vi "filled buttons.vi"(9 "control-level":string, 11 "Material-Scheme in":refnum<class "Material-Scheme.lvclass">) -> (1 "font color":u32(colorbox), 2 "colors array":cluster{"bg":u32, "fg":u32}[](array[cluster]))   [LabVIEW 2021, in "TSC Material Theme.lvlib" / "Material-Scheme.lvclass"]
doc: "application of the FILLED buttons coloring rules\n\nhttps://m3.material.io/components/buttons/specs#7b9ba06e-d393-491b-830e-ae3fe0816d4b\n\n<b>Code Developed By:</b> +\nDaniel Coons +\nTechnology Service Corporation +\nwww.tsc.com/atcs"
uses:
  Material-Scheme.lvclass
  Material-Scheme.lvclass/Material-Scheme.ctl
  <vilib>/Utility/colorconv.llb/Color to RGB.vi
  <vilib>/Utility/colorconv.llb/RGB to Color.vi
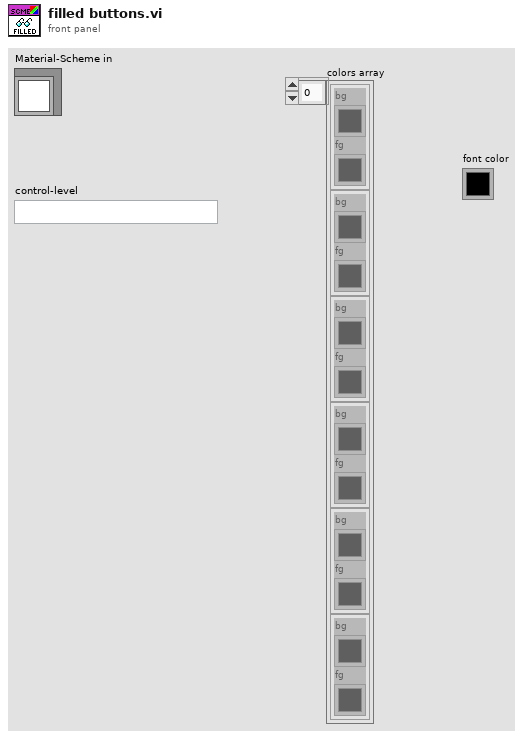
[diagram p1: front panel]
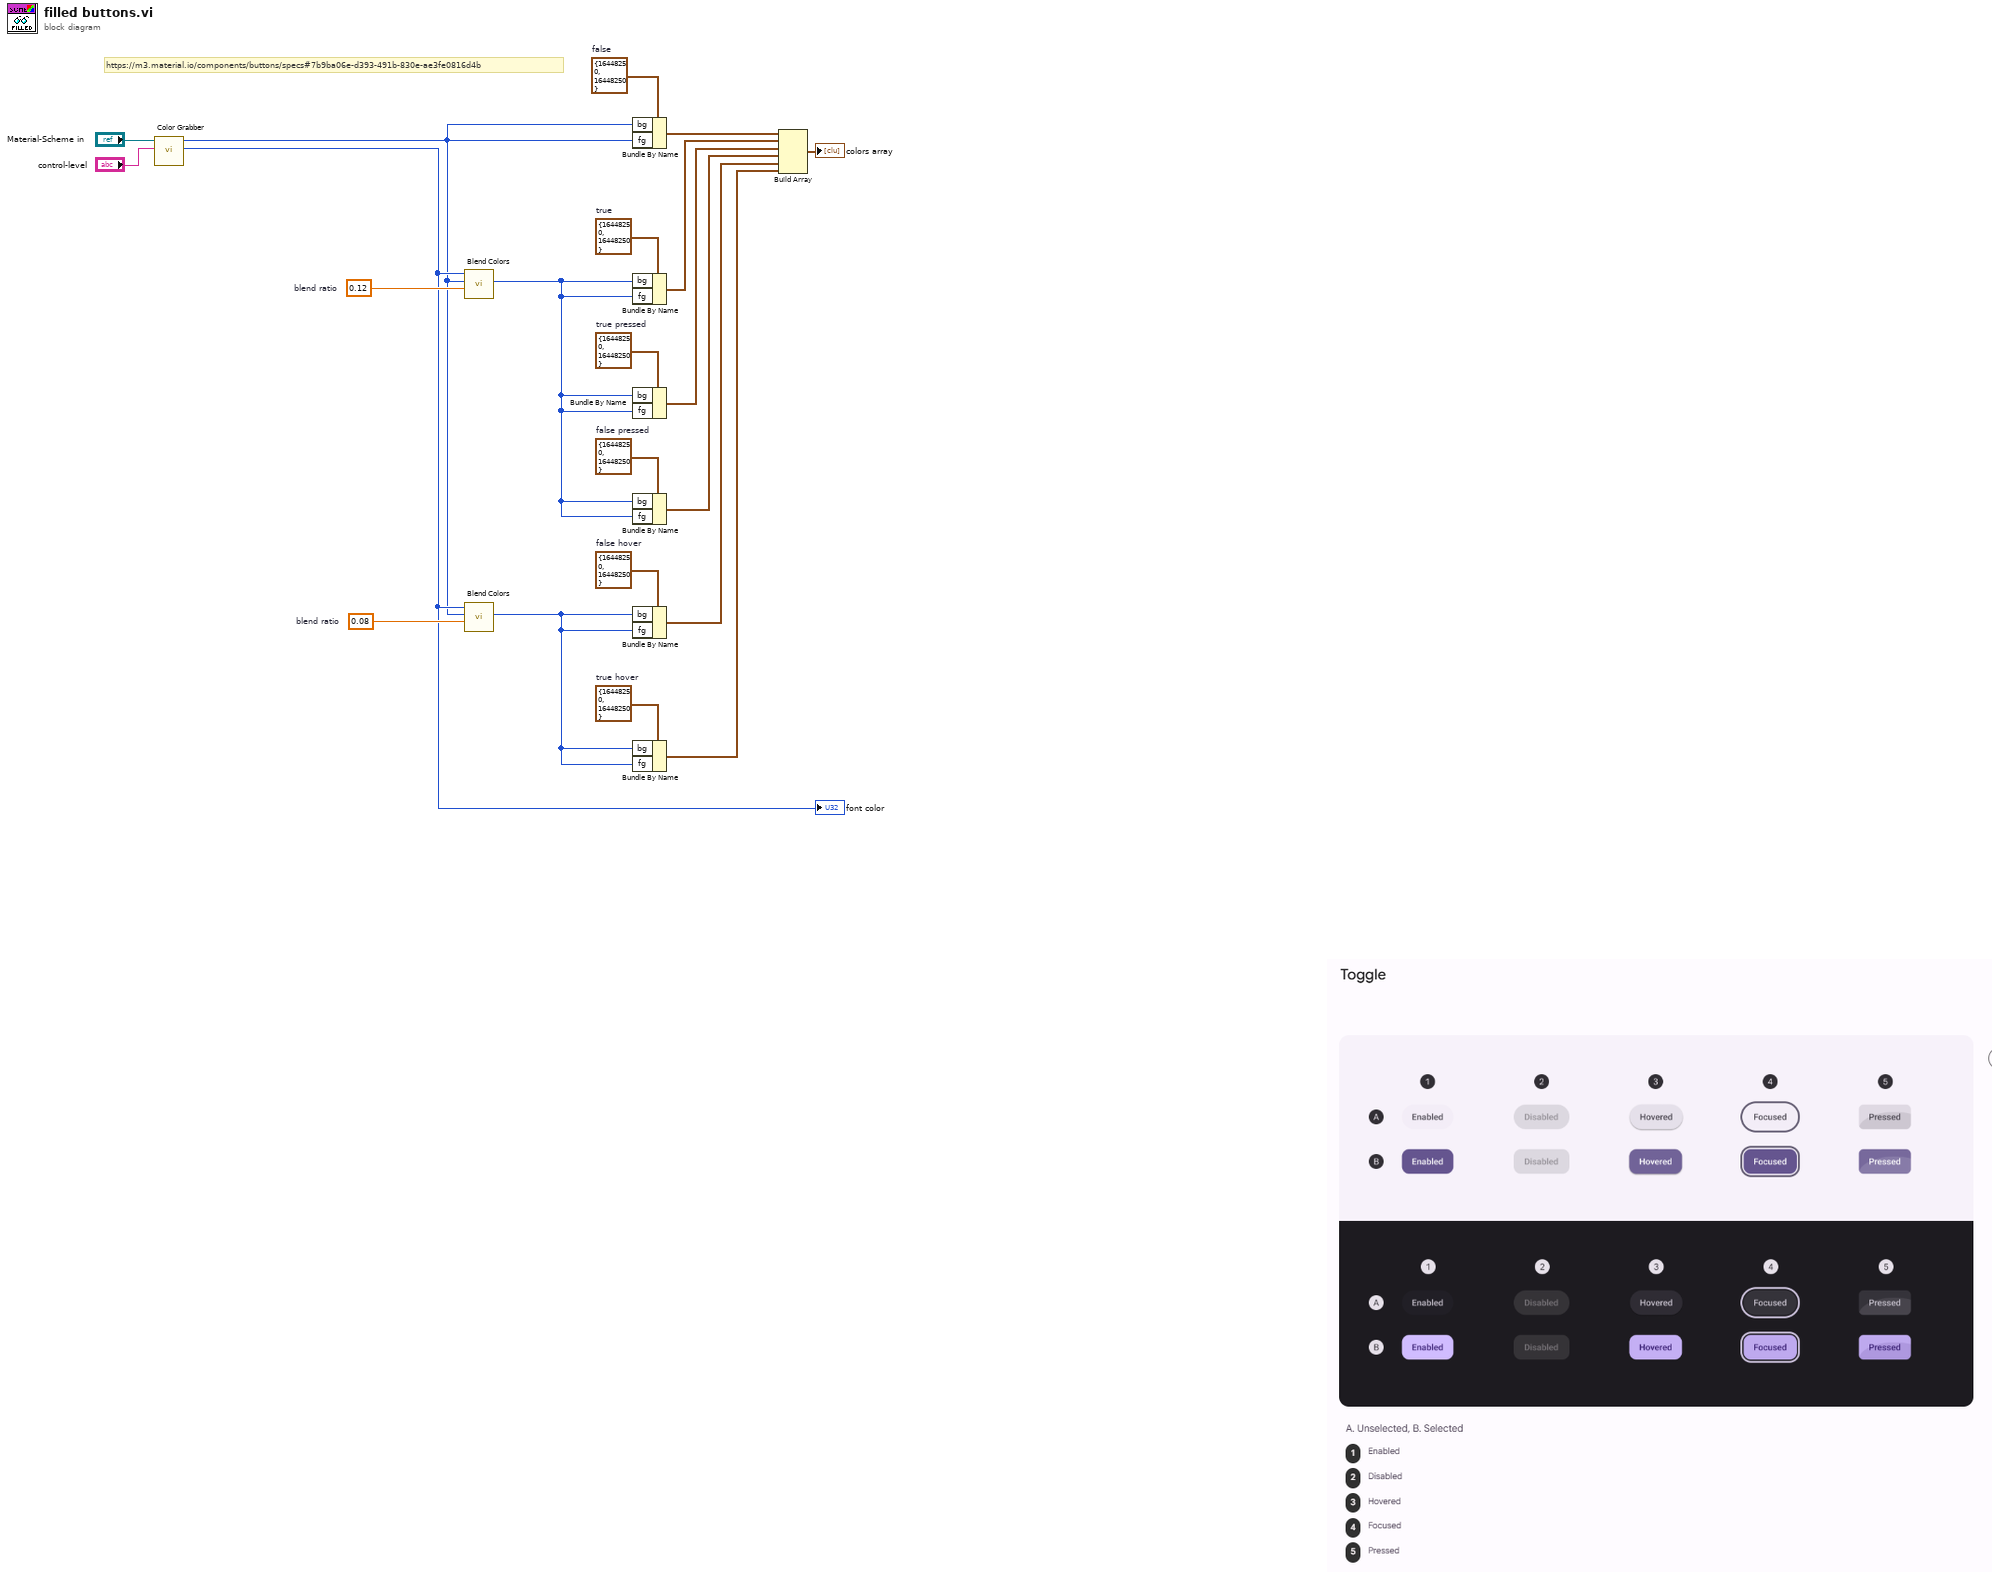
[diagram p0: block diagram]
diagram:
  w6 = 0.08  # blend ratio
  w7 = 0.12  # blend ratio
  w16 = cluster{"bg":u32, "fg":u32} {"bg"=16448250, "fg"=16448250}  # true hover
  w17 = cluster{"bg":u32, "fg":u32} {"bg"=16448250, "fg"=16448250}  # false hover
  w18 = cluster{"bg":u32, "fg":u32} {"bg"=16448250, "fg"=16448250}  # false pressed
  w19 = cluster{"bg":u32, "fg":u32} {"bg"=16448250, "fg"=16448250}  # true pressed
  w20 = cluster{"bg":u32, "fg":u32} {"bg"=16448250, "fg"=16448250}  # true
  w21 = cluster{"bg":u32, "fg":u32} {"bg"=16448250, "fg"=16448250}  # false
  # "https://m3.material.io/components/buttons/specs#7b9ba06e-d393-491b-830e-ae3fe0816d4b"
  n1 = call "Color Grabber.vi"("control-level"="control-level", "Material-Scheme in"="Material-Scheme in") -> ("onColor"=w4:u32, "color"=w3:u32)  [unwired: 3 in, 5 out]
  "font color" <- w4
  n2 = call "Blend Colors.vi"("blend ratio"=w7, "onColor"=w3, "Color"=w4) -> ("Modified Color"=w1:u32)  [unwired: 8 in]
  n3 = call "Blend Colors.vi"("blend ratio"=w6, "onColor"=w3, "Color"=w4) -> ("Modified Color"=w2:u32)  [unwired: 8 in]
  n4 = Bundle By Name(cluster=w21, "bg"=w3, "fg"=w3) -> (w15:cluster{"bg":u32, "fg":u32})
  n5 = Bundle By Name(cluster=w20, "bg"=w1, "fg"=w1) -> (w14:cluster{"bg":u32, "fg":u32})
  n6 = Bundle By Name(cluster=w19, "bg"=w1, "fg"=w1) -> (w13:cluster{"bg":u32, "fg":u32})
  n7 = Bundle By Name(cluster=w18, "bg"=w1, "fg"=w1) -> (w12:cluster{"bg":u32, "fg":u32})
  n8 = Bundle By Name(cluster=w17, "bg"=w2, "fg"=w2) -> (w11:cluster{"bg":u32, "fg":u32})
  n9 = Bundle By Name(cluster=w16, "bg"=w2, "fg"=w2) -> (w10:cluster{"bg":u32, "fg":u32})
  n10 = Build Array(w15, w14, w13, w12, w11, w10) -> (→"colors array":cluster{"bg":u32, "fg":u32}[])
